vi "Do.vi"(8 "error in (no error)":errorcluster, 10 "Actor in":refnum<class "Actor.lvclass">, 11 "SwitchOption Msg":refnum<class "SwitchOption Msg.lvclass">) -> (0 "error out":errorcluster, 2 "Actor out":refnum<class "Actor.lvclass">)   [LabVIEW 2015, in "Member_Actor.lvlib" / "SwitchOption Msg.lvclass"]
doc: "This VI delivers the message to the actor by calling the appropriate method(s) on the actor."
uses:
  SwitchOption Msg.lvclass
  <vilib>/ActorFramework/Actor/Actor.lvclass
  Member_Actor/Member_Actor.lvclass
  User_Actor/Member_Actor Messages/SwitchOption Msg/SwitchOption Msg.lvclass/SwitchOption Msg.ctl
  User_Actor/Member_Actor Messages/SwitchOption Msg/SwitchOption Msg.lvclass
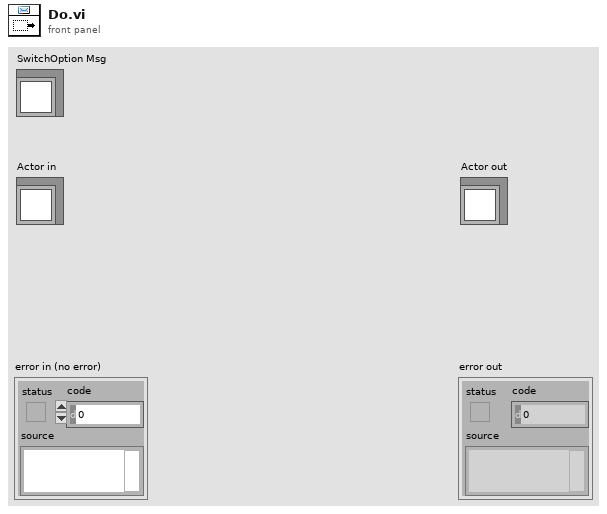
[diagram p1: front panel]
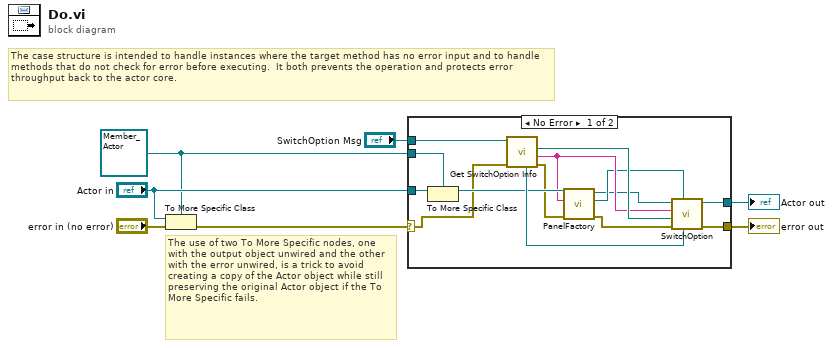
[diagram p0: block diagram]
diagram:
  w2 = refnum<class "Member_Actor.lvclass"> refnum ("Actor in")
  # "The use of two To More Specific nodes, one with the output object unwired and the other with the error unwired, is a trick to avoid creating a copy of the Actor object while still preserving the original Actor object if the To More Specific fails."
  # "The case structure is intended to handle instances where the target method has no error input and to handle methods that do not check for error before executing.  It both prevents the operation and protects error throughput back to the actor core."
  n1 = To More Specific Class(target class=w2, reference="Actor in", error in="error in (no error)") -> (error out=w6:errorcluster)  [unwired: 1 out]
  n2 = case shown="No Error" w6 {
    selector: w6 -> [w9 w23]
    tunnel: [w21 w23] -> w5
    tunnel: [w20 w22] -> w4
    tunnel: "Actor in" -> [w19 w22]
    tunnel: w2 -> [w18 _]
    tunnel: "SwitchOption Msg" -> [w17 _]
    frame No Error {
      n3 = To More Specific Class(target class=w18, reference=w19) -> (specific class reference=w14:refnum<class "Member_Actor.lvclass">)  [unwired: 1 in, 1 out]
      n4 = call "Get SwitchOption Info.vi"("error in (no error)"=w9, "SwitchOption Msg in"=w17) -> ("error out"=w8:errorcluster, "ThreadName(\"\")"=w13:string, "Base Path"=w16:path, "SubPanelRef"=w15:refnum<vi>)  [unwired: 5 in, 1 out]
      n5 = call-dynamic "PanelFactory.vi"("error in (no error)"=w8, "ThreadName(\"\")"=w13, "Member_Actor in"=w14) -> ("error out"=w10:errorcluster, "MemberPanel(Product)"=w12:refnum<class "MemberPanel.lvclass">, "Member_Actor out"=w11:refnum<class "Member_Actor.lvclass">)  [unwired: 6 in]
      n6 = call-dynamic "SwitchOption.vi"("SubPanelRef"=w15, "Panel Controller"=w12, "error in (no error)"=w10, "Base Path"=w16, "ThreadName(\"\")"=w13, "Member_Actor in"=w11) -> ("error out"=w21:errorcluster, "Member_Actor out"=w20:refnum<class "Member_Actor.lvclass">)  [unwired: 4 in]
    }
    frame Error {
      # "If type check fails, pass the original object out again."
    }
  }
  "error out" <- w5
  "Actor out" <- w4
